vi "4CHDAQ - Clear AO Channel.vi"(8 "error in":errorcluster, 11 "task/channels in":refnum<k21>) -> (0 "error out":errorcluster, 3 "task out":refnum<k21>)   [LabVIEW 2015]
uses:
  <vilib>/DAQmx/write.llb/DAQmx Write (Analog 1D DBL 1Chan NSamp).vi
  <vilib>/DAQmx/configure/timing.llb/DAQmx Timing (Sample Clock).vi
  <vilib>/DAQmx/miscellaneous.llb/DAQmx Fill In Error Info.vi
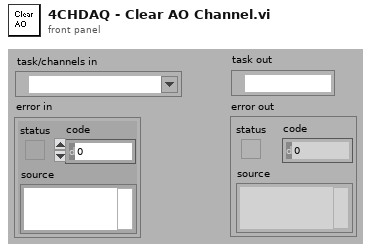
[diagram p1: front panel]
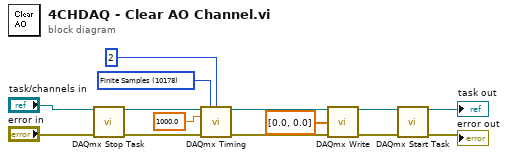
[diagram p0: block diagram]
diagram:
  w7 = 10178 items=["Finite Samples"=10178, "Continuous Samples"=10123, "Hardware Timed Single Point"=12522] ("sample mode")
  n1 = call <vilib>:"DAQmx Stop Task.vi"("task/channels in"="task/channels in", "error in"="error in") -> ("task out"=w2:refnum<k21>, "error out"=w1:errorcluster)  [unwired: 12 in]
  n2 = call-poly <vilib>:"DAQmx Timing.vi"("task/channels in"=w2, "sample mode"=w7, "samples per channel"=2, "rate"=1000.0, "error in"=w1) -> ("task out"=w4:refnum<k21>, "error out"=w3:errorcluster)  [unwired: 9 in]
  n3 = call-poly <vilib>:"DAQmx Write.vi"("task/channels in"=w4, "data"=dbl[] [0.0, 0.0], "error in"=w3) -> ("task out"=w14:refnum<k21>, "error out"=w13:errorcluster)  [unwired: 10 in, 1 out]
  n4 = call <vilib>:"DAQmx Start Task.vi"("task/channels in"=w14, "error in"=w13) -> ("task out"=→"task out":refnum<k21>, "error out"=→"error out":errorcluster)  [unwired: 12 in]
